vi "Parse Zone Data.vi"(10 "Zones":T1[](array[typedef]), 11 "JSONCluster in":T2) -> (3 "JSONCluster out":T2)   [LabVIEW 2015]
uses:
  Typedef/JSONCluster.ctl
  Typedef/Zone Data.ctl
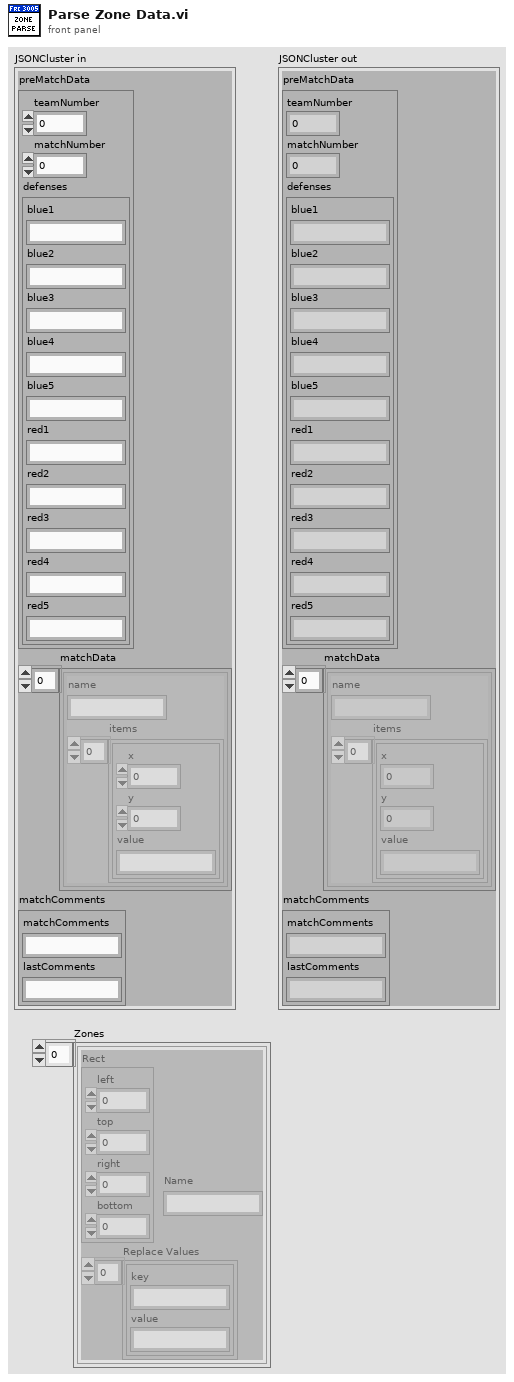
[diagram p1: front panel]
types:
  T1 = typedef "Zone Data.ctl" = cluster{"Rect":cluster{"left":i16, "top":i16, "right":i16, "bottom":i16}, "Replace Values":cluster{"key":string, "value":string}[], "Name":string}
  T2 = typedef "JSONCluster.ctl" = cluster{"preMatchData":cluster{"teamNumber":i32, "matchNumber":i32, "defenses":cluster{"blue1":string, "blue2":string, "blue3":string, "blue4":string, "blue5":string, "red1":string, "red2":string, "red3":string, "red4":string, "red5":string}}, "matchData":cluster{"name":string, "items":cluster{"x":i32, "y":i32, "value":string}[]}[], "matchComments":cluster{"matchComments":string, "lastComments":string}}
  T3 = cluster{"name":string, "items":cluster{"x":i32, "y":i32, "value":string}[]}[]
  T4 = cluster{"left":i16, "top":i16, "right":i16, "bottom":i16}
  T5 = cluster{"name":string, "items":cluster{"x":i32, "y":i32, "value":string}[]}
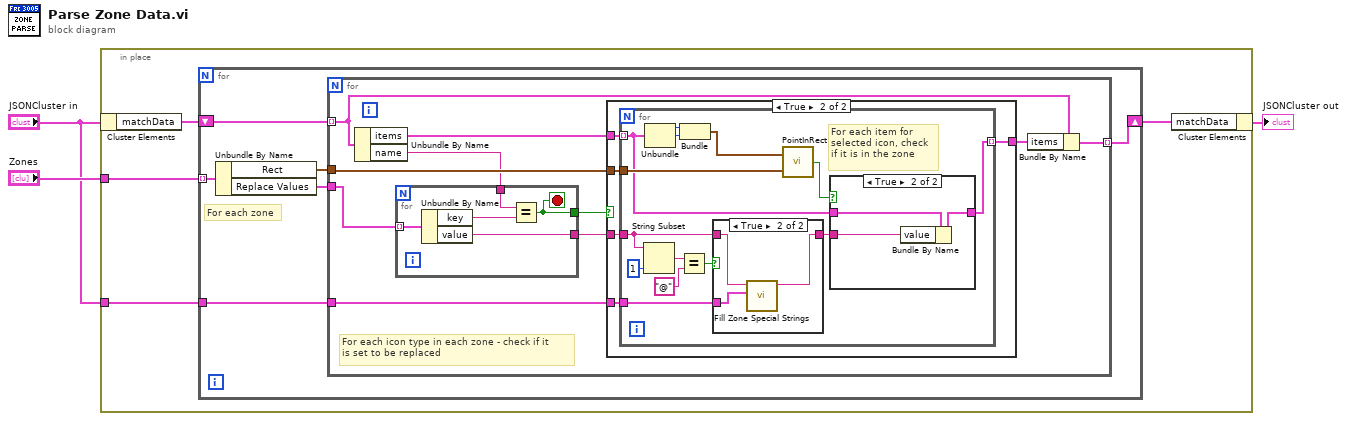
[diagram p0: block diagram]
diagram:
  n1 = in-place {
    in-place-border: "Zones" -> [w7]
    in-place-border: "JSONCluster in" -> [w4]
    n2 = in-place-cluster #1("JSONCluster in") -> ("matchData"=w6:T3)
    n3 = for {
      tunnel: w7 -> [w13] mode=indexing
      shift-right: [w9] -> w5
      shift-left: w6 -> [w12]
      tunnel: w4 -> [w8]
      # "For each zone"
      n4 = Unbundle By Name(w13) -> ("Rect"=w11:T4, "Replace Values"=w10:cluster{"key":string, "value":string}[])
      n5 = for {
        tunnel: w12 -> [w17] mode=indexing
        tunnel: w11 -> [w23]
        tunnel: w10 -> [w21]
        tunnel: [w15] -> w9 mode=indexing
        tunnel: w8 -> [w14]
        # "For each icon type in each zone - check if it \nis set to be replaced"
        n6 = Unbundle By Name(w17) -> ("items"=w22:cluster{"x":i32, "y":i32, "value":string}[], "name"=w20:string)
        n7 = for {
          tunnel: w21 -> [w56] mode=indexing
          tunnel: w20 -> [w55]
          tunnel: [w53] -> w19
          tunnel: [w52] -> w18
          stop <- w52 stop-if-true
          n8 = Unbundle By Name(w56) -> ("key"=w54:string, "value"=w53:string)
          n9 = Equal?(x=w55, y=w54) -> (x = y?=w52:bool)
        }
        n10 = case shown="True" w18 {
          tunnel: w23 -> [_ w29]
          tunnel: w22 -> [w24 w28]
          tunnel: w19 -> [_ w27]
          tunnel: [w24 w26] -> w16
          tunnel: w14 -> [_ w25]
          frame False {
          }
          frame True {
            n11 = for {
              tunnel: w29 -> [w43]
              tunnel: w28 -> [w38] mode=indexing
              tunnel: w27 -> [w31]
              tunnel: [w37] -> w26 mode=indexing
              tunnel: w25 -> [w32]
              # "For each item for \nselected icon, check\nif it is in the zone"
              n12 = String Subset(string=w31, length (rest)=1 ("length (rest)")) -> (substring=w35:string)  [unwired: 1 in]
              n13 = Unbundle(w38) -> ("x"=w42:i32, "y"=w41:i32)  [unwired: 1 out]
              n14 = Equal?(x=w35, y="@") -> (x = y?=w33:bool)
              n15 = Bundle("x"=w42, "y"=w41) -> (w40:cluster{"x":i32, "y":i32})  [unwired: 1 in]
              n16 = case shown="True" w33 {
                tunnel: w32 -> [_ w47]
                tunnel: w31 -> [w44 w46]
                tunnel: [w44 w45] -> w30
                frame False {
                }
                frame True {
                  n17 = call "Fill Zone Special Strings.vi"("JSONCluster in"=w47, "value in"=w46) -> ("replaced value"=w45:string)  [unwired: 9 in]
                }
              }
              n18 = call <vilib>:"PointInRect.vi"("rect"=w43, "point"=w40) -> ("pt in rect"=w39:bool)
              n19 = case shown="True" w39 {
                tunnel: w38 -> [w48 w51]
                tunnel: [w48 w50] -> w37
                tunnel: w30 -> [_ w49]
                frame False {
                }
                frame True {
                  n20 = Bundle By Name(cluster=w51, "value"=w49) -> (w50:cluster{"x":i32, "y":i32, "value":string})
                }
              }
            }
          }
        }
        n21 = Bundle By Name(cluster=w17, "items"=w16) -> (w15:T5)
      }
    }
    n22 = in-place-cluster #1("matchData"=w5) -> (→"JSONCluster out":T2)
  }
